vi "Line1004.vi"   [LabVIEW 2013]
uses:
  <vilib>/Heliosphere Research LLC/Advanced Plotting Toolkit/api_plotting/LineProperties.ctl
  <vilib>/Heliosphere Research LLC/Advanced Plotting Toolkit/properties/Line.ctl
  <vilib>/Heliosphere Research LLC/Advanced Plotting Toolkit/properties/Line_Style.ctl
  <vilib>/Heliosphere Research LLC/Advanced Plotting Toolkit/typedefs/PlotColor.ctl
  <vilib>/Heliosphere Research LLC/Advanced Plotting Toolkit/properties/Marker.ctl
  <vilib>/Heliosphere Research LLC/Advanced Plotting Toolkit/properties/Marker_Style.ctl
  <vilib>/Heliosphere Research LLC/Advanced Plotting Toolkit/properties/Display.ctl
  <vilib>/Heliosphere Research LLC/Advanced Plotting Toolkit/Advanced Plotting Toolkit.lvlib
types:
  T1 = typedef "Advanced Plotting Toolkit.lvlib/LineProperties.ctl" = cluster{"Line":T2, "Marker":T5, "Display":T7}
  T2 = typedef "Advanced Plotting Toolkit.lvlib/Line.ctl" = cluster{"Style":T3, "Color":T4, "Width":sgl}
  T3 = typedef "Advanced Plotting Toolkit.lvlib/Line_Style.ctl" = enum16{"Automatic", "Solid", "Dashed", "Dotted", "Dash-dot", "Invisible"}
  T4 = typedef "Advanced Plotting Toolkit.lvlib/PlotColor.ctl" = u32
  T5 = typedef "Advanced Plotting Toolkit.lvlib/Marker.ctl" = cluster{"Style":T6, "Color":T4, "Size":dbl}
  T6 = typedef "Advanced Plotting Toolkit.lvlib/Marker_Style.ctl" = enum16{"Automatic", "Circle", "Square", "Triangle", "Diamond", "Star", "Invisible"}
  T7 = typedef "Advanced Plotting Toolkit.lvlib/Display.ctl" = cluster{"Alpha":dbl, "Z Order":dbl}
  T8 = typedef "Advanced Plotting Toolkit.lvlib/PlotID.ctl" = i32
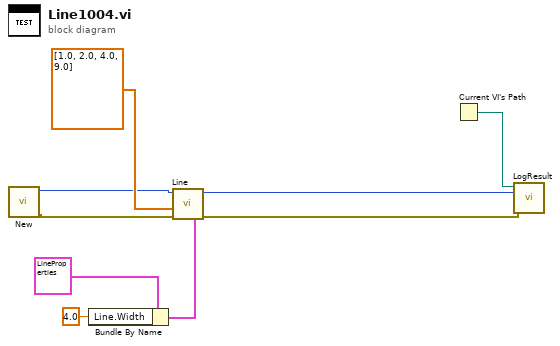
[diagram p0: block diagram]
diagram:
  n1 = call <vilib>:"New.vi"() -> ("error out"=w5:errorcluster, "Plot ID"=w7:T8)  [unwired: 10 in]
  n2 = Bundle By Name(cluster=T1 {"Line"={"Style"=enum."Automatic", "Color"=2147483647, "Width"=nan}, "Marker"={"Style"=enum."Automatic", "Color"=2147483647, "Size"=nan}, "Display"={"Alpha"=nan, "Z Order"=nan}} ("Line Plot Properties"), "Line.Width"=sgl 4.0) -> (w2:T1)
  n3 = call <vilib>:"Line.vi"("Properties"=w2, "error in (no error)"=w5, "Y Data"=dbl[] [1.0, 2.0, 4.0, 9.0], "Plot ID"=w7) -> ("error out"=w4:errorcluster, "Plot ID out"=w6:T8)  [unwired: 6 in]
  n4 = Current VI's Path() -> (path=w9:path)
  n5 = call "LogResult.vi"("Test Result"=w4, "Test Artifact"=w6, "VI Path"=w9) -> ()  [unwired: 9 in]
